vi "Receive Message via UDP.vi"(8 "error in":errorcluster, 9 "timeout ms (25000)":i32=25000, 11 "Local Port":u16) -> (0 "error out":errorcluster, 3 "Message":T1)   [LabVIEW 2021]
uses:
  Message.ctl
  Action.ctl
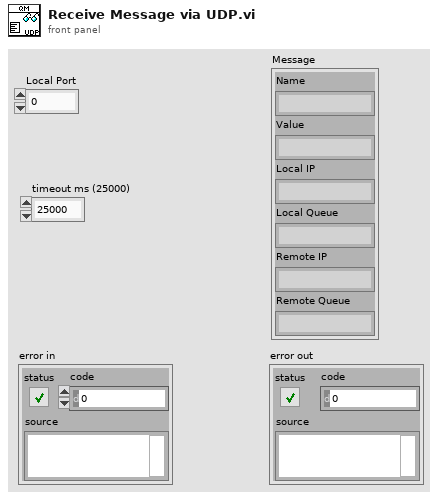
[diagram p1: front panel]
types:
  T1 = typedef "Message.ctl" = cluster{"Name":string, "Value":string, "Local IP":string, "Local Queue":string, "Remote IP":string, "Remote Queue":string}
  T2 = typedef "Action.ctl" = enum16{"Get", "Close"}
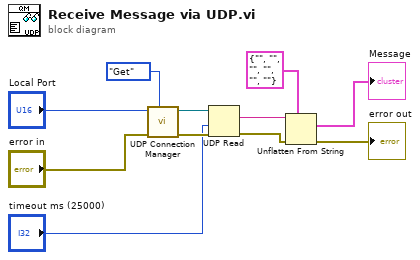
[diagram p0: block diagram]
diagram:
  n1 = call "UDP Connection Manager.vi"("Action"=Action."Get", "error in (no error)"="error in", "UDP Port"="Local Port") -> ("error out"=w5:errorcluster, "connection ID out"=w4:refnum<k16>)  [unwired: 7 in]
  n2 = UDP Read(connection ID=w4, timeout ms (25000)="timeout ms (25000)", 8:w5) -> (data out=w10:string, error out=w8:errorcluster)  [unwired: 1 in, 3 out]
  n3 = Unflatten From String(type=T1 {"Name"="", "Value"="", "Local IP"="", "Local Queue"="", "Remote IP"="", "Remote Queue"=""} ("Message"), binary string=w10, error in (no error)=w8) -> (value=→"Message":T1, error out=→"error out":errorcluster)  [unwired: 2 in, 1 out]
